vi "Draw Filled Poly (Greyscale).vi"(4 "Point Type (Default: Any)":T1, 6 "OpenCV Line Type (Default LINE_8)":T4=enum."LINE_8", 7 "Colour":u8=255, 8 "error in (no error)":errorcluster, 10 "Points":T2[](array[typedef]), 11 "Greyscale Image in":T3) -> (0 "error out":errorcluster, 3 "Greyscale Image":T3)   [LabVIEW 2020, in "image.lvlib"]
doc: "Draw a filled polynomial based on the given points."
uses:
  image.lvlib
  Line Type.ctl
  Greyscale Image.ctl
  common/Image Point (Integer).ctl
  Fill-Poly Points Type.ctl
  e24a04ad-8575-4d64-b8af-da4c51ecb9cd.vi
  <vilib>/Utility/error.llb/Error Cluster From Error Code.vi
  common/common.lvlib
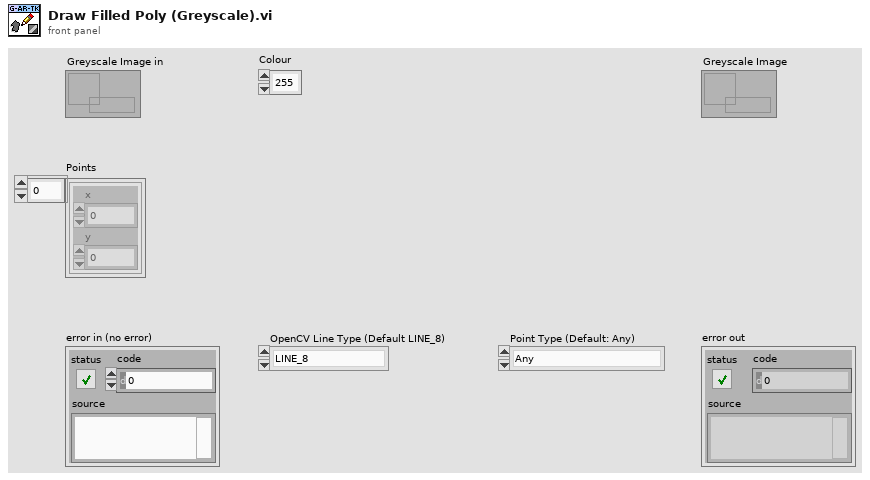
[diagram p1: front panel]
types:
  T1 = typedef "image.lvlib/Fill-Poly Points Type.ctl" = enum8{"Any", "Convex Only"}
  T2 = typedef "common.lvlib/Image Point (Integer).ctl" = cluster{"x":i32, "y":i32}
  T3 = typedef "image.lvlib/Greyscale Image.ctl" = refnum<data-value>
  T4 = typedef "image.lvlib/Line Type.ctl" = enum8{"FILLED", "LINE_4", "LINE_8", "LINE_AA"}
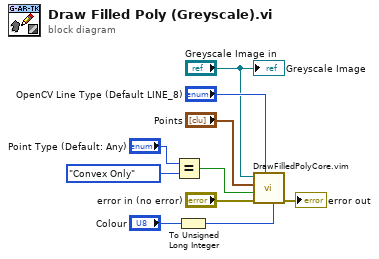
[diagram p0: block diagram]
diagram:
  n1 = Equal?(x="Point Type (Default: Any)", y=Fill-Poly_Points_Type."Convex Only") -> (x = y?=w2:bool)
  n2 = To Unsigned Long Integer(number="Colour") -> (unsigned 32bit integer=w6:u32)
  n3 = call "DrawFilledPolyCore.vim"("Colour"=w6, "OpenCV Line Type"="OpenCV Line Type (Default LINE_8)", "error in (no error)"="error in (no error)", "Is Convex"=w2, "Points"="Points", "Src"="Greyscale Image in") -> ("error out"=→"error out":errorcluster)  [unwired: 5 in]
  "Greyscale Image" <- "Greyscale Image in"
